vi "ShowErrorOscVI.vi"(8 "error in (no error)":errorcluster, 11 "Oscilloscope in":refnum<class "Oscilloscope.lvclass">) -> (0 "error out":errorcluster, 3 "Oscilloscope out":refnum<class "Oscilloscope.lvclass">)   [LabVIEW 2018, in "Oscilloscope.lvclass"]
uses:
  Oscilloscope.lvclass
  C:/Users/Sergey Denisov/Documents/REPS/TRANCON/Classes/GeneralFunctionality/GeneralFunctionality.lvclass
  GeneralFunctionality/GeneralFunctionality.lvclass/GeneralFunctionality.ctl
  GeneralFunctionality/GeneralFunctionality.lvclass
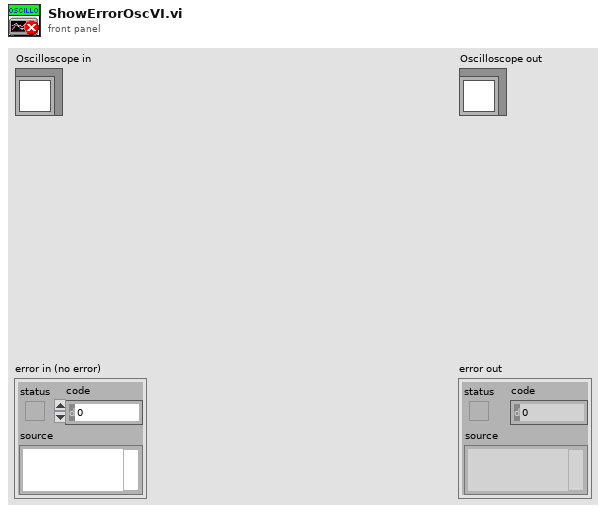
[diagram p1: front panel]
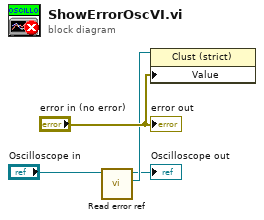
[diagram p0: block diagram]
diagram:
  n1 = call "Read error ref.vi"("GeneralFunctionality in"="Oscilloscope in") -> ("error"=w3:refnum<vi>, "GeneralFunctionality out"=→"Oscilloscope out":refnum<class "Oscilloscope.lvclass">)  [unwired: 8 in, 1 out]
  n2 = property class="Clust (strict)"(reference=w3, "Value"="error in (no error)") -> ()  [unwired: 1 in, 2 out]
  "error out" <- "error in (no error)"
